vi "Read AutoCal Password.vi"(8 "error in":errorcluster) -> (0 "error out":errorcluster, 3 "Password":string)   [LabVIEW 2015]
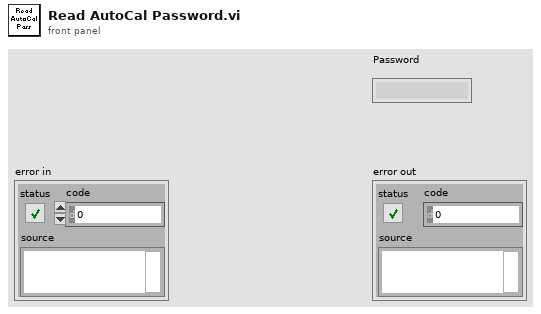
[diagram p1: front panel]
types:
  T1 = enum16{"open", "replace", "create", "open or create", "replace or create", "replace or create with confirmation"}
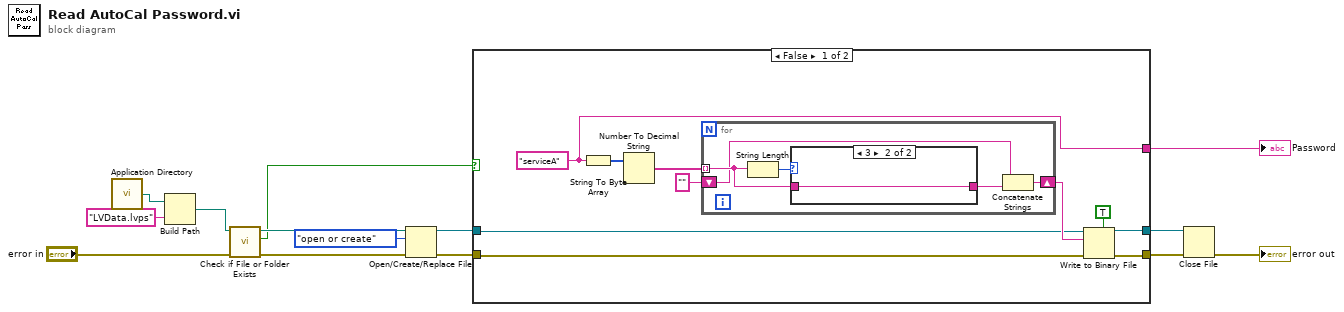
[diagram p0: block diagram]
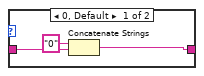
[diagram p2: hidden frame]
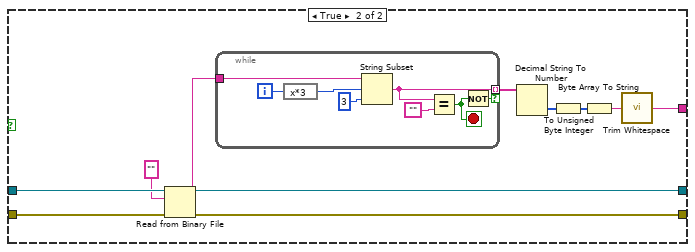
[diagram p3: hidden frame]
diagram:
  n1 = call <vilib>:"Application Directory.vi"() -> ("Application Directory"=w10:path)
  n2 = Build Path(base path=w10, name or relative path="LVData.lvps") -> (appended path=w7:path)
  n3 = call <vilib>:"Check if File or Folder Exists.vi"("error in (no error)"="error in", "path"=w7) -> ("error out"=w8:errorcluster, "file or folder exists?"=w4:bool, "dup path"=w6:path)  [unwired: 7 in]
  n4 = Open/Create/Replace File(file path (use dialog)=w6, error in=w8, operation (0:open)=T1."open or create") -> (refnum out=w14:refnum<file>, error out=w13:errorcluster)  [unwired: 3 in, 1 out]
  n5 = case shown="False" w4 {
    tunnel: w14 -> [w17 w44]
    tunnel: w13 -> [w16 w43]
    tunnel: [w15 w38] -> w12
    tunnel: [w19 w37] -> w3
    tunnel: [w18 w34] -> w1
    frame False {
      w15 = "serviceA" ("string")
      n6 = String To Byte Array(string=w15) -> (unsigned byte array=w20:u8[])
      n7 = Number To Decimal String(number=w20) -> (decimal integer string=w21:string[])  [unwired: 1 in]
      n8 = for {
        tunnel: w21 -> [w28] mode=indexing
        shift-right: [w26] -> w23
        shift-left: "" -> [w25]
        n9 = String Length(string=w28) -> (length=w29:i32)
        n10 = case shown="3" w29 {
          tunnel: w28 -> [w31 w33]
          tunnel: [w30 w33] -> w27
          frame 0, Default {
            n11 = Concatenate Strings("0" ("string"), w31) -> (w30:string)
          }
          frame 3 {
          }
        }
        n12 = Concatenate Strings(w25, w27) -> (w26:string)
      }
      n13 = Write to Binary File(file (use dialog)=w17, data=w23, error in=w16, 5:TRUE ("prepend array or string size? (T)")) -> (refnum out=w18:refnum<file>, error out=w19:errorcluster)  [unwired: 2 in, 1 out]
    }
    frame True {
      n14 = Read from Binary File(5:"" ("data"), 8:w43, 11:w44) -> (0:w37:errorcluster, 2:w41:string, 3:w34:refnum<file>)  [unwired: 3 in, 1 out]
      n15 = while {
        tunnel: w41 -> [w52]
        tunnel: [w47] -> w40 mode=indexing if=w45
        i -> [w51]
        stop <- w46 stop-if-true
        n16 = expression code="x*3"(w51) -> (w50:i32)
        n17 = String Subset(string=w52, offset (0)=w50, length (rest)=3 ("length (rest)")) -> (substring=w47:string)
        n18 = Equal?(x=w47, y="") -> (x = y?=w46:bool)
        n19 = Not(x=w46) -> (.not. x?=w45:bool)
      }
      n20 = Decimal String To Number(string=w40) -> (number=w36:i32[])  [unwired: 2 in, 1 out]
      n21 = To Unsigned Byte Integer(number=w36) -> (unsigned 8bit integer=w35:u8[])
      n22 = Byte Array To String(unsigned byte array=w35) -> (string=w39:string)
      n23 = call <vilib>:"Trim Whitespace.vi"("string"=w39) -> ("trimmed string"=w38:string)  [unwired: 1 in]
    }
  }
  "Password" <- w12
  n24 = Close File(refnum=w1, error in=w3) -> (error out=→"error out":errorcluster)  [unwired: 1 out]
